vi "Read Spectrum Data.vi"(8 "error in (no error)":errorcluster, 11 "VISA resource name":refnum<visa-resource-name>) -> (0 "error out":errorcluster, 1 "Spectra":i16[][](array[numeric]), 2 "Wavelength (nm)":dbl[](array[numeric]), 3 "VISA resource name out":refnum<visa-resource-name>, 5 "Time Stamp":dbl format="%#_20f")   [LabVIEW 2015, in "Micron Optics sm130.lvlib"]
doc: "Displays the spectral data for the channel selected in Configure Channel.vi. Timestamp and wavelength in nm are also displayed."
uses:
  Micron Optics sm130.lvlib
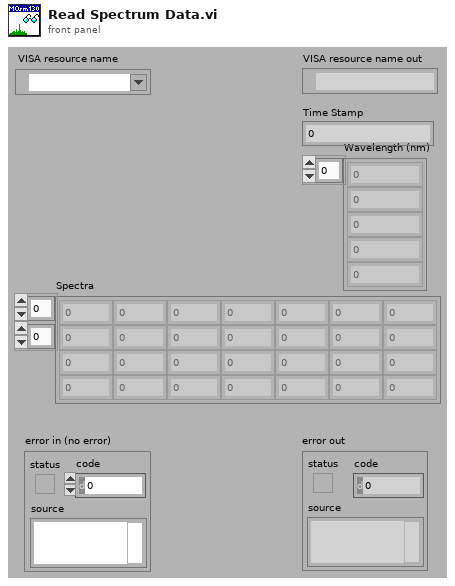
[diagram p1: front panel]
types:
  T1 = cluster{"Full Spectrum Radix":u8, "Firmware Version":u8, "Primary Fan":bool, "Secondary Fan":bool, "Switch Position":u8, "MUX":u8, "Trigger Mode":u8, "Operating Mode":u8, "Data Serial Number":u32, "Time Stamp":dbl, "Buffer (%)":u8, "MUX Level":u8}
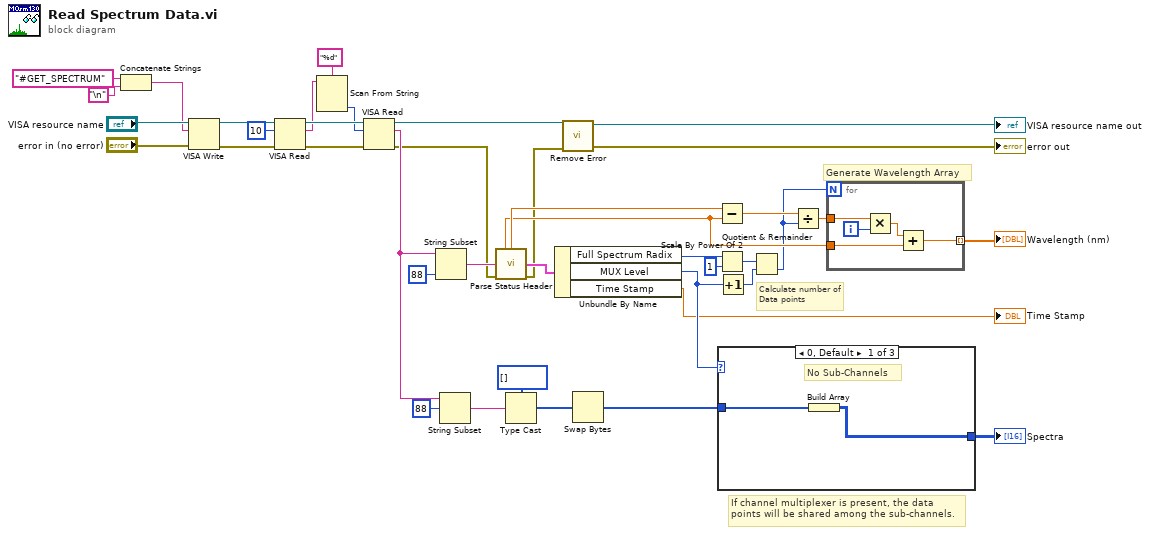
[diagram p0: block diagram]
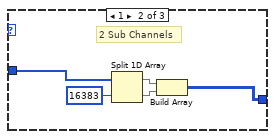
[diagram p2: hidden frame]
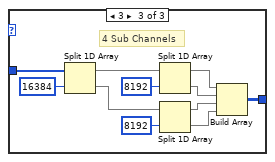
[diagram p3: hidden frame]
diagram:
  # "If channel multiplexer is present, the data points will be shared among the sub-channels."
  # "Calculate number of Data points"
  # "Generate Wavelength Array"
  n1 = Concatenate Strings("#GET_SPECTRUM" ("string"), "\n") -> (w28:string)
  n2 = VISA Write(VISA resource name="VISA resource name", write buffer=w28, error in (no error)="error in (no error)") -> (VISA resource name out=w34:refnum<visa-resource-name>, error out=w33:errorcluster)  [unwired: 1 out]
  n3 = VISA Read(VISA resource name=w34, byte count=u32 10, error in (no error)=w33) -> (VISA resource name out=w40:refnum<visa-resource-name>, read buffer=w37:string, error out=w39:errorcluster)  [unwired: 1 out]
  n4 = Scan From String(format string="%d", input string=w37) -> (output 1=w35:i32)  [unwired: 3 in, 3 out]
  n5 = VISA Read(VISA resource name=w40, byte count=w35, error in (no error)=w39) -> (VISA resource name out=w8:refnum<visa-resource-name>, read buffer=w24:string, error out=w3:errorcluster)  [unwired: 1 out]
  n6 = String Subset(string=w24, length (rest)=88 ("length (rest)")) -> (substring=w26:string)  [unwired: 1 in]
  n7 = String Subset(string=w24, offset (0)=88) -> (substring=w12:string)  [unwired: 1 in]
  n8 = call "Parse Status Header.vi"("Status Header In"=w26, "error in (no error)"=w3) -> ("Full Spectrum Starting Wavelength (nm)"=w14:dbl, "Full Spectrum Ending Wavelength (nm)"=w22:dbl, "Status"=w23:T1, "error out"=w2:errorcluster)  [unwired: 7 in, 3 out]
  n9 = Type Cast(type=i16[] [], x=w12) -> (*(type *) &x=w10:i16[])
  n10 = Unbundle By Name(w23) -> ("Full Spectrum Radix"=w21:u8, "MUX Level"=w17:u8, "Time Stamp"=→"Time Stamp":dbl)
  n11 = call "Remove Error.vi"("error in (no error)"=w2, "VISA resource name"=w8) -> ("error out"=→"error out":errorcluster, "VISA resource name out"=→"VISA resource name out":refnum<visa-resource-name>)  [unwired: 8 in]
  n12 = Swap Bytes(anything=w10) -> (byte swapped=w9:i16[])
  n13 = Subtract(x=w22, y=w14) -> (x-y=w16:dbl)
  n14 = Scale By Power Of 2(n=w21, x=u16 1) -> (x*2^n=w19:u16)
  n15 = Increment(x=w17) -> (x+1=w18:u8)
  n16 = case shown="0, Default" w17 {
    tunnel: w9 -> [w42 w47 w56]
    tunnel: [w41 w43 w48] -> w1
    frame 0, Default {
      # "No Sub-Channels"
      n17 = Build Array(w42) -> (w41:i16[][])
    }
    frame 1 {
      # "2 Sub Channels"
      n18 = Split 1D Array(array=w47, index=16383) -> (first subarray=w45:i16[], second subarray=w44:i16[])
      n19 = Build Array(w45, w44) -> (w43:i16[][])
    }
    frame 3 {
      # "4 Sub Channels"
      n20 = Split 1D Array(array=w56, index=16384) -> (first subarray=w58:i16[], second subarray=w57:i16[])
      n21 = Split 1D Array(array=w58, index=8192) -> (first subarray=w52:i16[], second subarray=w51:i16[])
      n22 = Split 1D Array(array=w57, index=8192) -> (first subarray=w50:i16[], second subarray=w49:i16[])
      n23 = Build Array(w52, w51, w50, w49) -> (w48:i16[][])
    }
  }
  "Spectra" <- w1
  n24 = Quotient & Remainder(x=w19, y=w18) -> (floor(x/y)=w13:u16)  [unwired: 1 out]
  n25 = Divide(x=w16, y=w13) -> (x/y=w15:dbl)
  n26 = for {
    N: w13 -> [_]
    tunnel: w15 -> [w63]
    tunnel: w14 -> [w60]
    tunnel: [w59] -> w5 mode=indexing
    i -> [w62]
    n27 = Multiply(x=w63, y=w62) -> (x*y=w61:dbl)
    n28 = Add(x=w61, y=w60) -> (x+y=w59:dbl)
  }
  "Wavelength (nm)" <- w5
